vi "ni579x Initialize EEPROM (poly).vi"   [LabVIEW 2013]
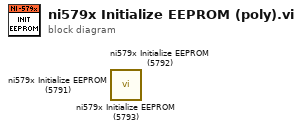
[diagram p0: block diagram]
diagram:
  n1 = call <instrlib>:"ni579x Initialize EEPROM (5793).vi"() -> ()  [unwired: 14 in, 2 out]
  n2 = call <instrlib>:"ni579x Initialize EEPROM (5792).vi"() -> ()  [unwired: 14 in, 2 out]
  n3 = call <instrlib>:"ni579x Initialize EEPROM (5791).vi"() -> ()  [unwired: 14 in, 2 out]
